vi "2013_01_03 Pre-Clinical Motor.vi"(9 "data":waveform(dbl)[](array[waveform]), 10 "File Path":path, 11 "cluster":T1) -> (0 "Final Out":dynamicdata(graph), 3 "Motor Typedef Out":T2={"Fail"=FALSE, "RPM"=0, "Supply (V)"=0.0, "Time"=1.0, "Counter"=0.0, "Torque (mNm)"=0.0, "Electrical (W)"=0.0, "Motor Eff"=0.0, "Mechanical (W)"=0.0, "Supply (W)"=0.0, "ESC Eff"=0.0} {"ESC Eff" format="%#_3g%%"; "Supply (W)" format="%.3f"; "Mechanical (W)" format="%.3f"; "Motor Eff" format="%#_3g%%"; "Electrical (W)" format="%.3f"; "Torque (mNm)" format="%.3f"; "Time" format="%<%H:%M:%S>t"; "Supply (V)" format="%.2f"})   [LabVIEW 2013]
uses:
  Pre-Clinical Type Def.ctl
  <vilib>/express/express shared/transition.llb/Dynamic To Waveform Array.vi
  <vilib>/express/express signal manip/GetorSetDDTAttributes/Set DDT Attributes/SetT0.vi
  <vilib>/express/express shared/transition.llb/Waveform Array To Dynamic.vi
  <vilib>/express/express signal manip/GetorSetDDTAttributes/Set DDT Attributes/Set DDT Properties.xnode
panel:
  in  "error in (no error)":errorcluster
  out "error out":errorcluster
  out "Saving Data":bool
  # "Stopped"
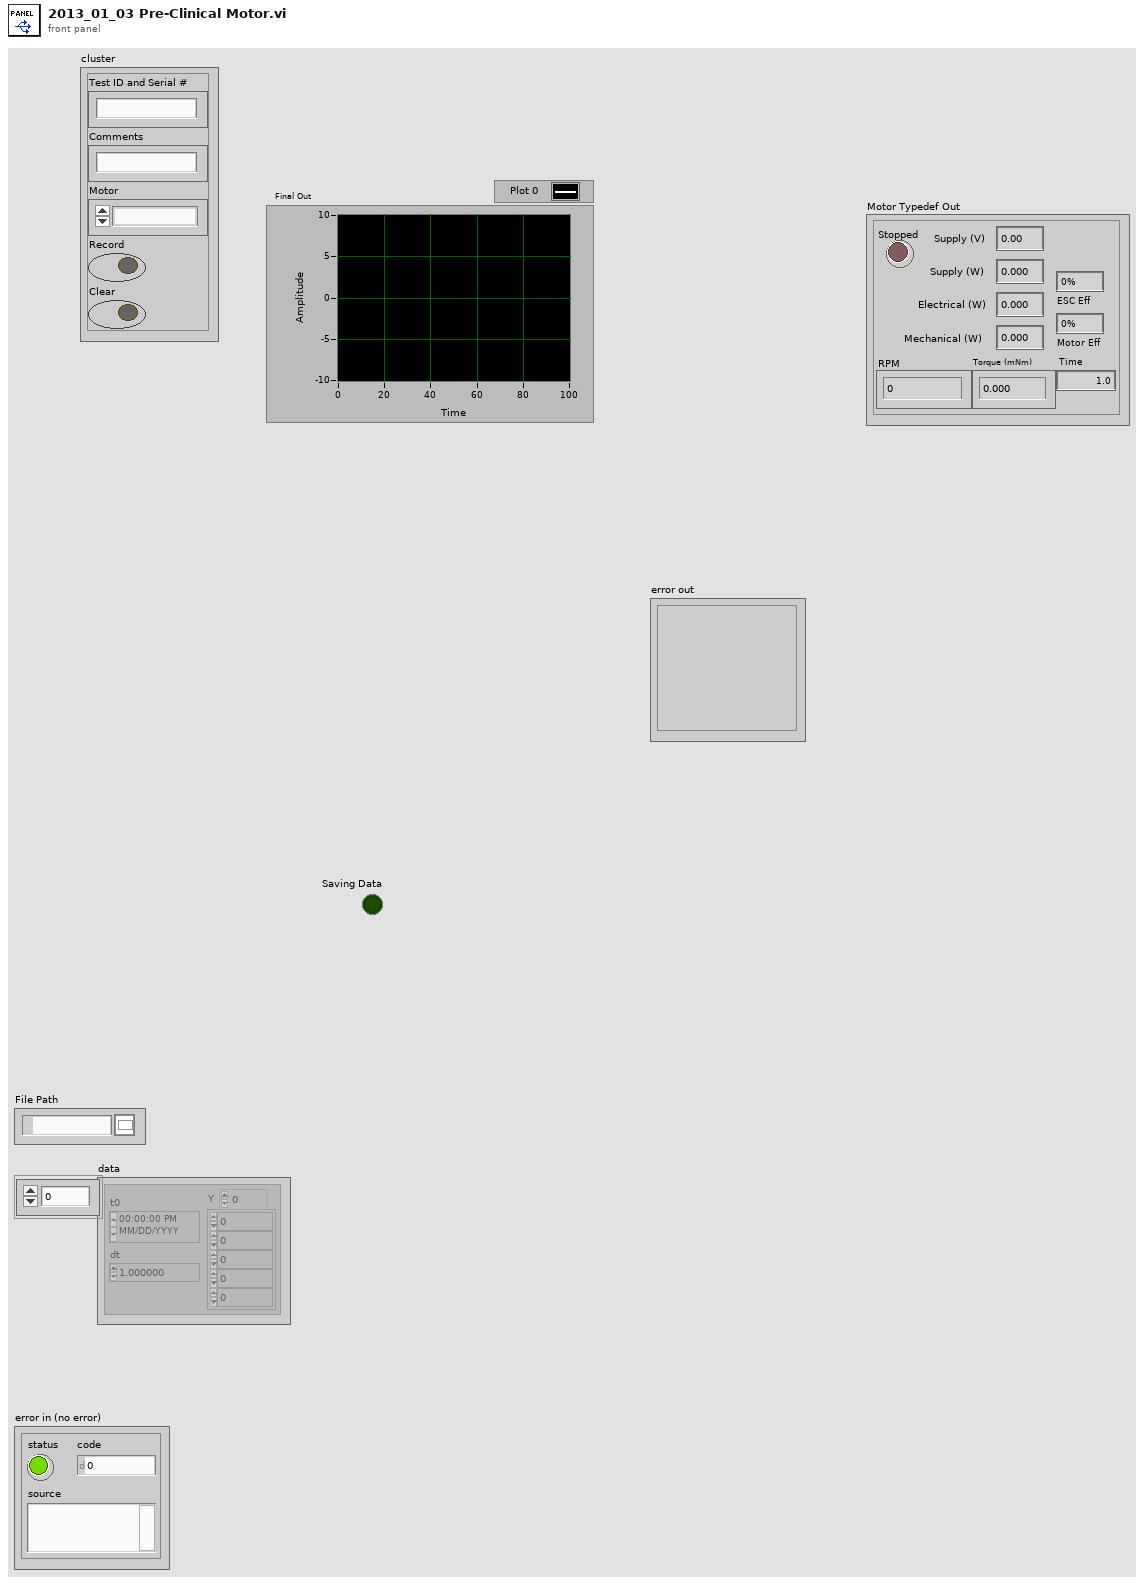
[diagram p1: front panel]
types:
  T1 = cluster{"Test ID and Serial #":string, "Comments":string, "Motor":enum16{"", "Maxon EC6 6V", "Maxon EC4 6V", "FH 0620 6V", "FH 0620 12V", "FH 0427 6V K2540"}, "Record":bool, "Clear":bool}
  T2 = typedef "Pre-Clinical Type Def.ctl" = cluster{"Fail":bool, "RPM":u64, "Supply (V)":dbl, "Time":dbl, "Counter":dbl, "Torque (mNm)":dbl, "Electrical (W)":dbl, "Motor Eff":dbl, "Mechanical (W)":dbl, "Supply (W)":dbl, "ESC Eff":dbl}
  T3 = enum16{"", "Maxon EC6 6V", "Maxon EC4 6V", "FH 0620 6V", "FH 0620 12V", "FH 0427 6V K2540"}
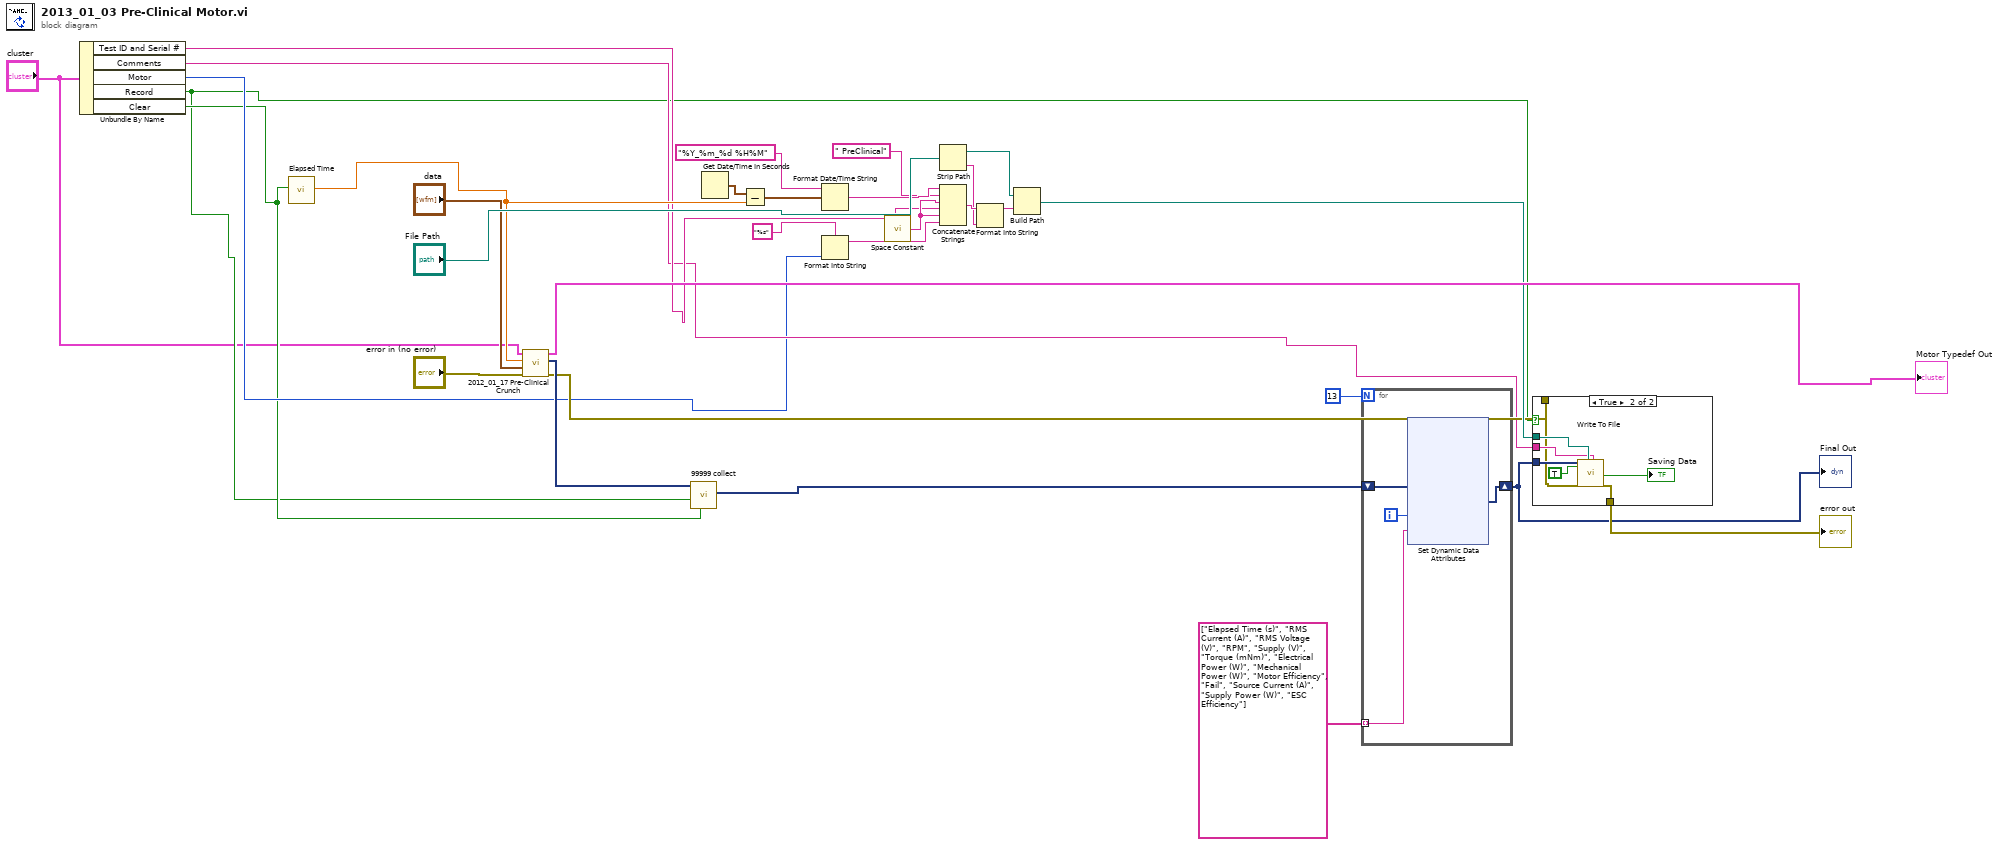
[diagram p0: block diagram]
diagram:
  n1 = Unbundle By Name("cluster") -> ("Test ID and Serial #"=w6:string, "Comments"=w5:string, "Motor"=w4:T3, "Record"=w2:bool, "Clear"=w3:bool)
  n2 = call "Elapsed Time"("Reset"=w3) -> ("Elapsed Time (s)"=w26:dbl)  [unwired: 11 in, 7 out]
  n3 = call "2012_01_17 Pre-Clinical Crunch.vi"("error in (no error)"="error in (no error)", "data"="data", "Elapsed Time (s)"=w26, "cluster"="cluster") -> ("error out"=w10:errorcluster, "Dynamic Data Type"=w19:dynamicdata, "Motor Out"=→"Motor Typedef Out":T2)  [unwired: 5 in]
  n4 = call "99999 collect"("Reset"=w3, "Enable"=w2, "Signals"=w19) -> ("Collected Signals"=w9:dynamicdata)  [unwired: 7 in, 1 out]
  n5 = Get Date/Time In Seconds() -> (seconds since 1Jan1904=w16:timestamp)
  n6 = Subtract(x=w16, y=w26) -> (x-y=w15:timestamp)
  n7 = Format Date/Time String(time format string (%c)="%Y_%m_%d %H%M", seconds (now)=w15) -> (date/time string=w8:string)  [unwired: 1 in]
  n8 = Format Into String(format string="%s", w4) -> (resulting string=w13:string)  [unwired: 2 in, 1 out]
  n9 = call <vilib>:"Space Constant.vi"() -> ("String"=w11:string)
  n10 = Strip Path(path="File Path") -> (stripped path=w21:path, name=w22:string)
  n11 = Concatenate Strings(w8, " PreClinical" ("string"), w11, w6, w11, w13) -> (w23:string)
  n12 = Format Into String(initial string=w23, w22) -> (resulting string=w20:string)  [unwired: 2 in, 1 out]
  n13 = Build Path(base path=w21, name or relative path=w20) -> (appended path=w24:path)
  n14 = for {
    N: 13 -> [_]
    tunnel: string[] ["Elapsed Time (s)", "RMS Current (A)", "RMS Voltage (V)", "RPM", "Supply (V)", "Torque (mNm)", "Electrical Power (W)", "Mechanical Power (W)", "Motor Efficiency", "Fail", "Source Current (A)", "Supply Power (W)", "ESC Efficiency"] ("appended array") -> [w33] mode=indexing
    shift-right: [w34] -> w27
    shift-left: w9 -> [w32]
    i -> [w35]
    n15 = xnode "Set Dynamic Data Attributes"("Signals In"=w32, "Signal Index"=w35, "Signal Name"=w33) -> ("Signals Out"=w34:dynamicdata)  [unwired: 1 in, 1 out]
  }
  "Final Out" <- w27
  n16 = case shown="True" w2 {
    tunnel: w27 -> [_ w56]
    tunnel: w24 -> [_ w55]
    tunnel: w5 -> [_ w52]
    tunnel: [w49 w51] -> w30
    tunnel: w10 -> [w49 w50]
    frame False {
    }
    frame True {
      n17 = call "Write To File"("Signals"=w56, "Reset"=TRUE, "error in (no error)"=w50, "Filename"=w55, "Comment"=w52) -> ("Saving Data"=→"Saving Data":bool, "error out"=w51:errorcluster)  [unwired: 12 in, 1 out]
    }
  }
  "error out" <- w30
